vi "CalcNewValue.vi"(4 "Dead rule":i32[](array[numeric])=[3], 6 "Live rule":i32[](array[numeric])=[2, 3], 9 "j":i32=69, 10 "i":i32=69, 11 "Main Board":T1[][](array[typedef])=array70x70[4900 elements]) -> (2 "New value":T1)   [LabVIEW 2020]
doc: "Calc new value of one elementar cell."
uses:
  Ctrls/ElementalCell.ctl
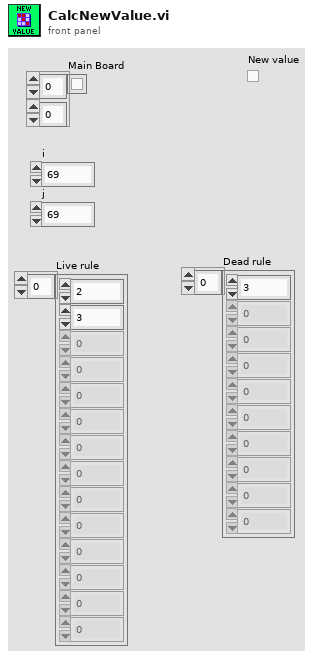
[diagram p1: front panel]
types:
  T1 = typedef "ElementalCell.ctl" = bool
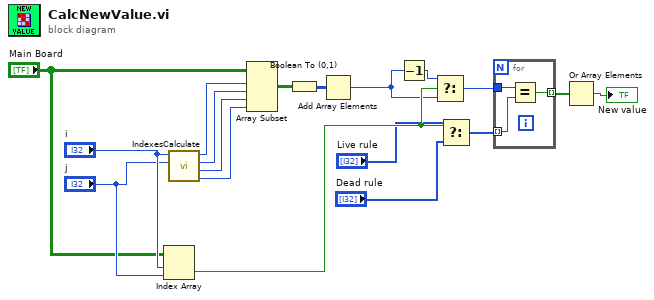
[diagram p0: block diagram]
diagram:
  n1 = Index Array(array="Main Board", index (row)="i", index (col)="j") -> (element=w12:T1)
  n2 = call "IndexesCalculate.vi"("j"="j", "i"="i") -> ("j_l"=w15:i32, "j*"=w16:i32, "i_l"=w17:i32, "i*"=w18:i32)  [unwired: 6 in]
  n3 = Array Subset(array="Main Board", index (row)=w18, length (row)=w17, index (col)=w16, length (col)=w15) -> (w10:T1[][])
  n4 = Boolean To (0,1)(Boolean=w10) -> (0, 1=w11:i16[][])
  n5 = Add Array Elements(numeric array=w11) -> (sum=w9:i16)
  n6 = Decrement(x=w9) -> (x-1=w3:i16)
  n7 = Select(t=w3, s=w12, f=w9) -> (s? t:f=w2:i16)
  n8 = Select(t="Live rule", s=w12, f="Dead rule") -> (s? t:f=w4:i32[])
  n9 = for {
    tunnel: w2 -> [w21]
    tunnel: [w20] -> w5 mode=indexing
    tunnel: w4 -> [w19] mode=indexing
    n10 = Equal?(x=w21, y=w19) -> (x = y?=w20:bool)
  }
  n11 = Or Array Elements(Boolean array=w5) -> (logical OR=→"New value":bool)
